vi "DataSummarizer.vi"() -> ()   [LabVIEW 2025]
uses:
  Controls/State.ctl
  ff876046-9b6a-4137-aed5-b25abd0cf997.vi
  <vilib>/Array/Sort 2D Array - Pop Stack.vi
  <vilib>/Array/Sort 2D Array - Push Stack.vi
  <vilib>/Utility/file.llb/Write Delimited Spreadsheet (string).vi
panel:
  out "output array":string[][](array[string])
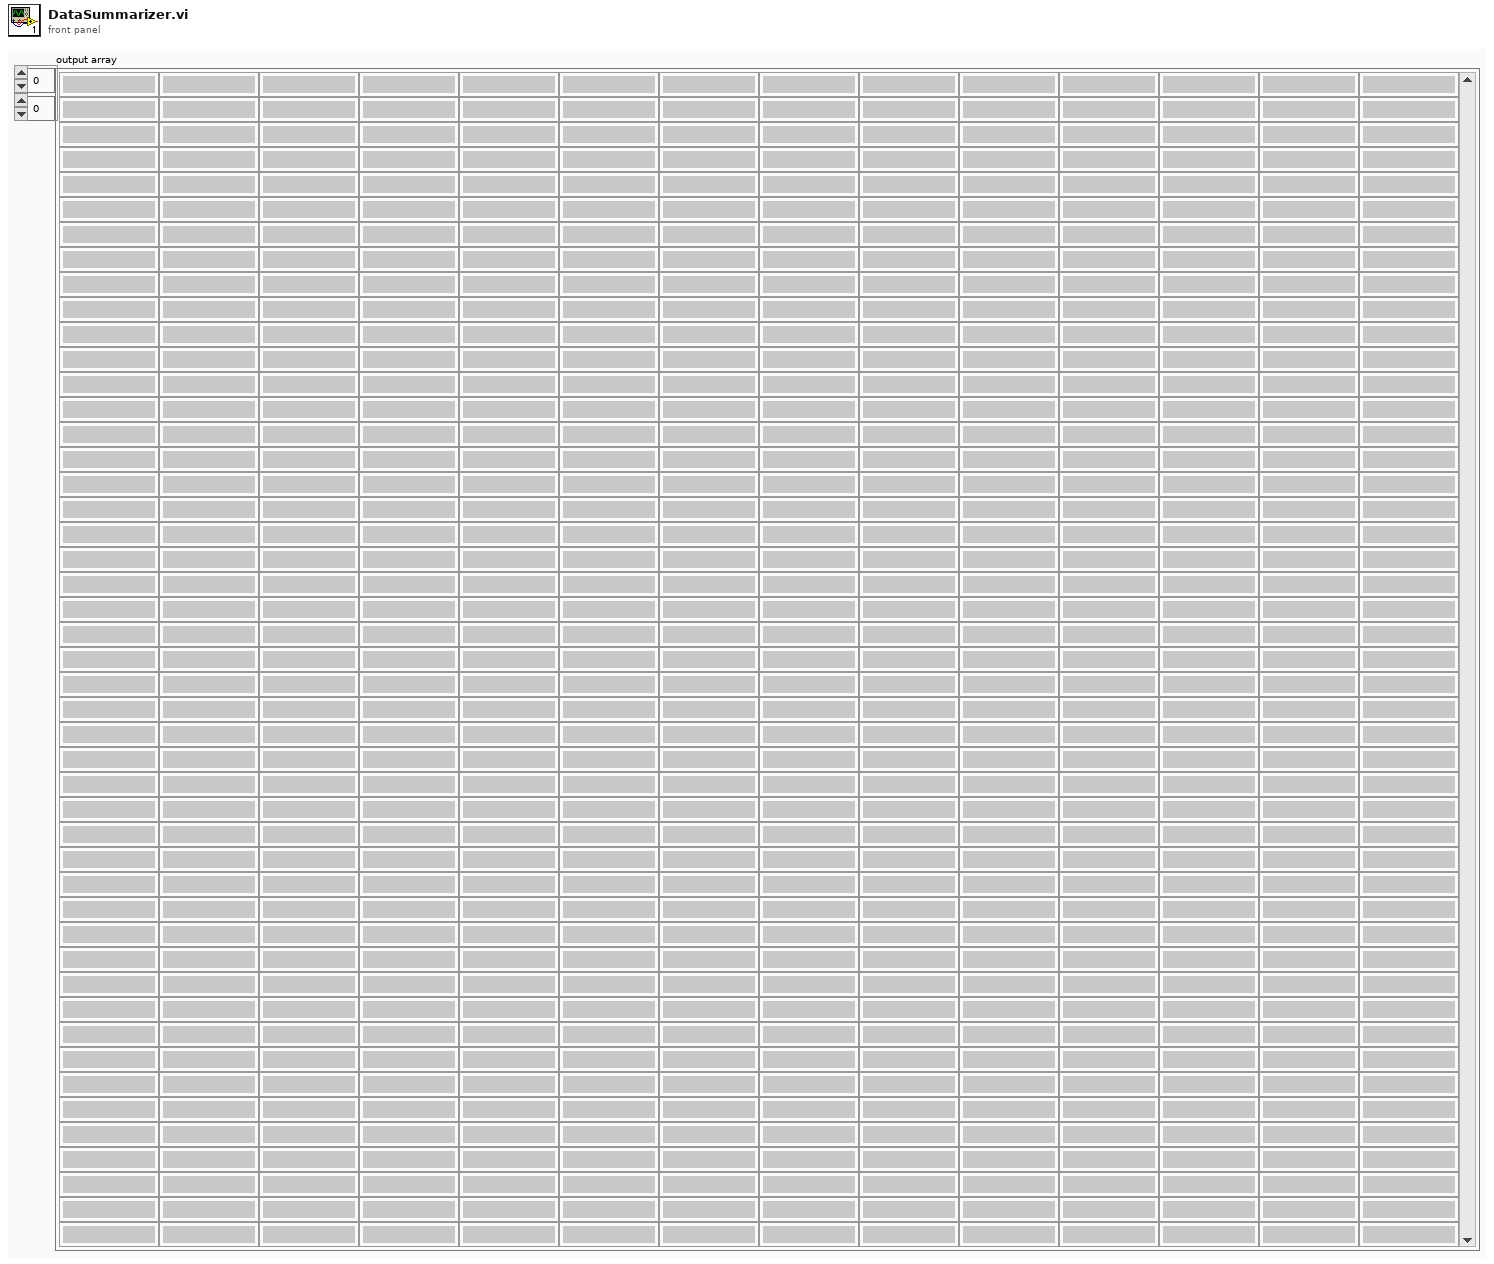
[diagram p1: front panel]
types:
  T1 = typedef "State.ctl" = enum16{"Init", "Idle", "Analyze", "End"}
  T2 = typedef "Dependand_Variables.ctl" = cluster{"Task Completion Times":dbl[], "TCT mean":dbl, "Error rate":i32, "Overshoots":i32[], "Overshoot  mean":dbl, "Overshoot times":dbl[], "Overshoot times mean":dbl, "targets out?":bool[], "No targets selected?":bool[], "No targets selected":i32}
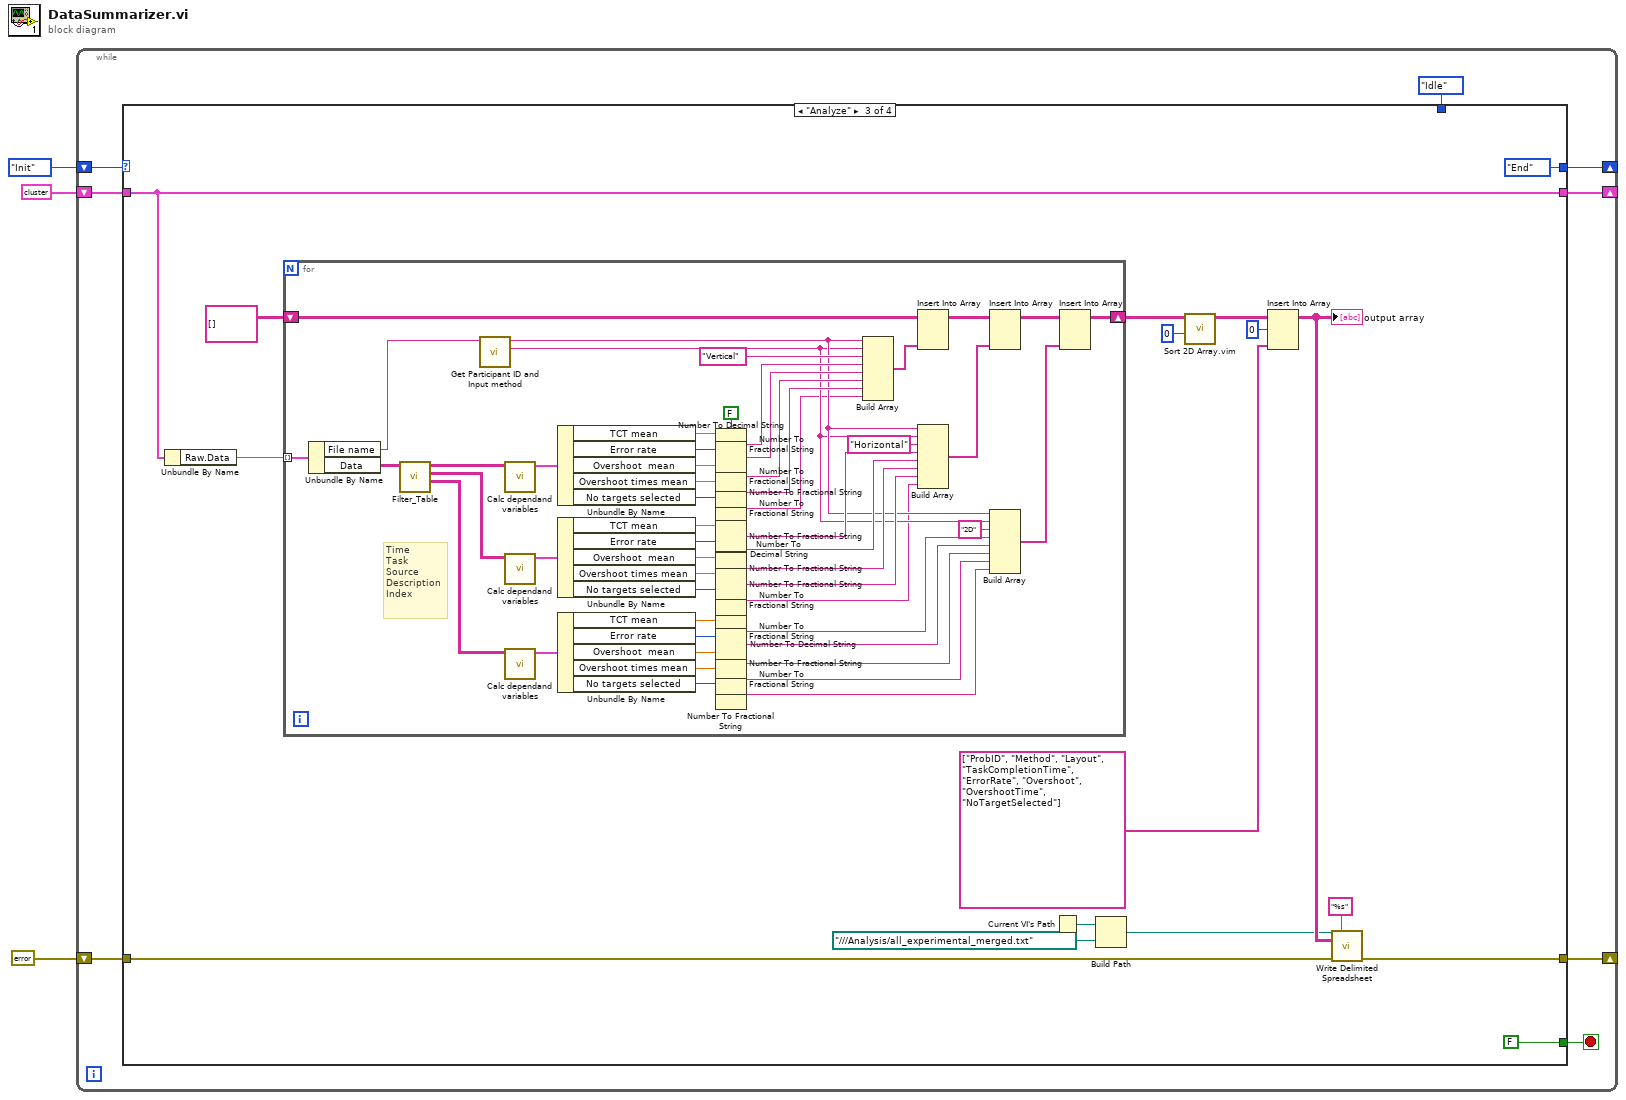
[diagram p0: block diagram]
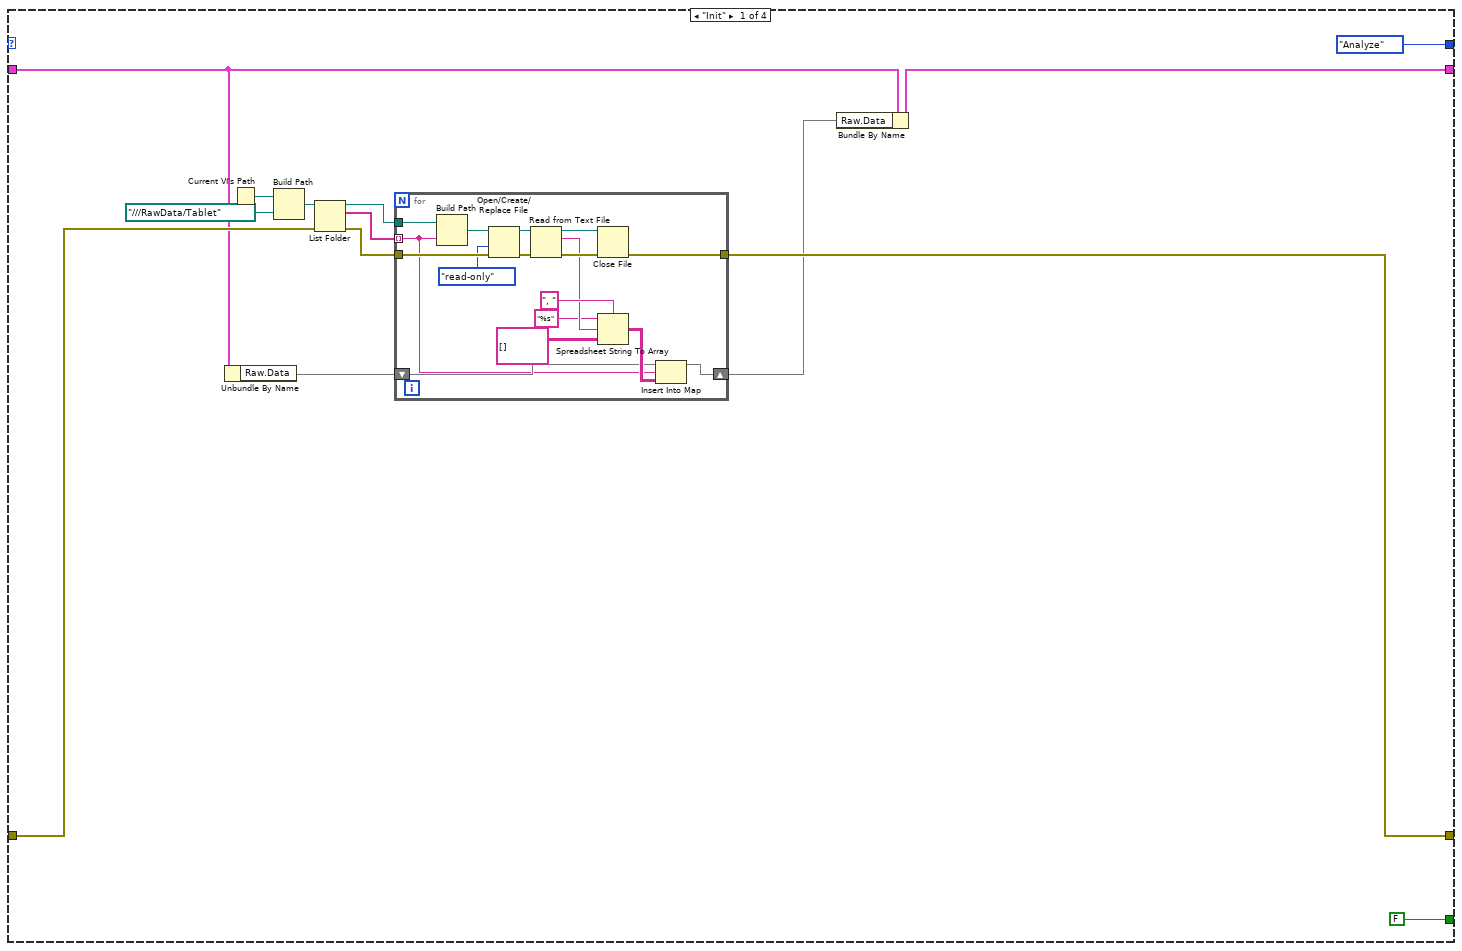
[diagram p2: hidden frame]
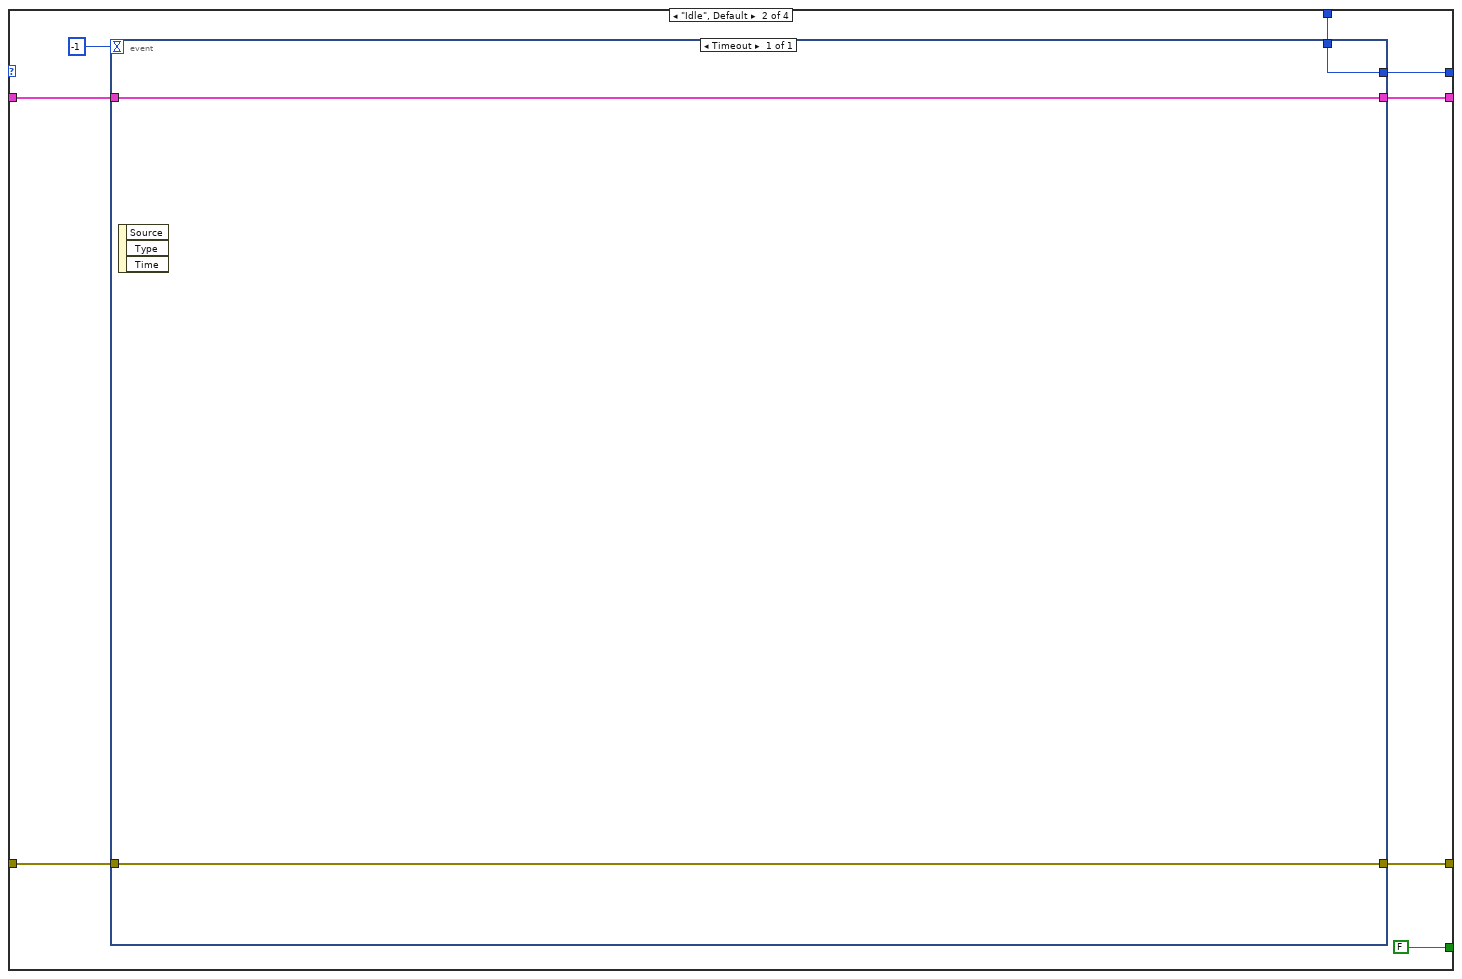
[diagram p3: hidden frame]
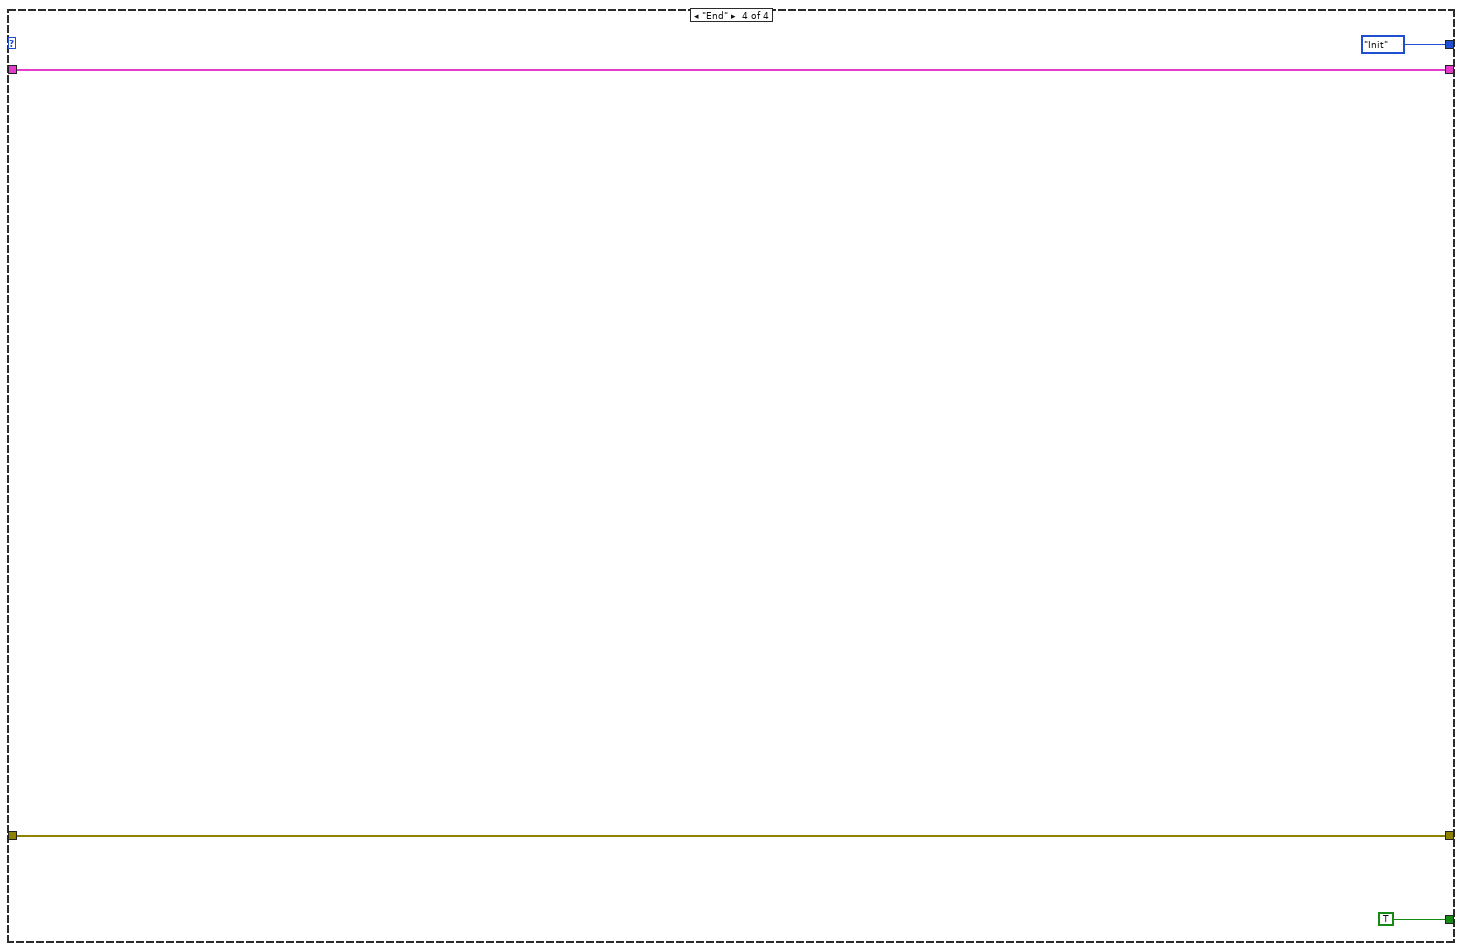
[diagram p4: hidden frame]
diagram:
  n1 = while {
    shift-right: [w9] -> _
    shift-left: errorcluster {"status"=FALSE, "code"=0, "source"=""} ("error constant") -> [w10]
    shift-right: [w8] -> _
    shift-left: State."Init" -> [w11]
    shift-right: [w5] -> _
    shift-left: cluster{"Raw.Data":map{string, string[][]}} {"Raw.Data"={}} -> [w6]
    stop <- w4 stop-if-true
    n2 = case shown="\"Analyze\"" w11 {
      tunnel: w10 -> [w22 w49 w58 w126]
      tunnel: [w21 w50 w57 w126] -> w9
      tunnel: [State."Analyze" w47 State."End" State."Init"] -> w8
      tunnel: State."Idle" -> [_ w46 _ _]
      tunnel: w6 -> [w18 w44 w69 w123]
      tunnel: [w19 w45 w69 w123] -> w5
      tunnel: [FALSE FALSE FALSE TRUE] -> w4
      frame "Init" {
        n3 = Unbundle By Name(w18) -> ("Raw.Data"=w17:map{string, string[][]})
        n4 = Current VI's Path() -> (path=w14:path)
        n5 = Build Path(base path=w14, name or relative path=path "../../../RawData/Tablet") -> (appended path=w12:path)
        n6 = List Folder(path=w12, error in=w22) -> (path out=w24:path, filenames=w25:string[], error out=w23:errorcluster)  [unwired: 2 in, 1 out]
        n7 = for {
          tunnel: w23 -> [w42]
          tunnel: w24 -> [w37]
          tunnel: w25 -> [w26] mode=indexing
          tunnel: [w30] -> w21
          shift-right: [w27] -> w16
          shift-left: w17 -> [w28]
          n8 = Build Path(base path=w37, name or relative path=w26) -> (appended path=w36:path)
          n9 = Open/Create/Replace File(file path (use dialog)=w36, error in=w42, access (0:read/write)=enum16{"read/write", "read-only", "write-only"}."read-only") -> (refnum out=w41:refnum<file>, error out=w40:errorcluster)  [unwired: 3 in, 1 out]
          n10 = Read from Text File(file (use dialog)=w41, error in=w40) -> (refnum out=w39:refnum<file>, text=w33:string, error out=w38:errorcluster)  [unwired: 2 in, 1 out]
          n11 = Close File(refnum=w39, error in=w38) -> (error out=w30:errorcluster)  [unwired: 1 out]
          n12 = Spreadsheet String To Array(delimiter (Tab)=", ", format string="%s", spreadsheet string=w33, array type (2D Dbl)=string[][] []) -> (array=w29:string[][])
          n13 = Insert Into Map(map in=w28, key=w26, value=w29) -> (map out=w27:map{string, string[][]})  [unwired: 2 out]
        }
        n14 = Bundle By Name(cluster=w18, "Raw.Data"=w16) -> (w19:cluster{"Raw.Data":map{string, string[][]}})
      }
      frame "Idle", Default {
        n15 = event shown="[0] Timeout" {
          selector: _ -> [_]
          dyn-events: _ -> [_]
          timeout: -1 -> [_]
          tunnel: [w53] -> w50
          tunnel: w49 -> [w53]
          tunnel: [w52] -> w47
          tunnel: w46 -> [w52]
          tunnel: [w51] -> w45
          tunnel: w44 -> [w51]
          event Timeout {
            n16 = event-data() -> ()  [unwired: 1 in, 3 out]
          }
        }
      }
      frame "Analyze" {
        n17 = Unbundle By Name(w69) -> ("Raw.Data"=w68:map{string, string[][]})
        n18 = for {
          tunnel: w68 -> [w120] mode=indexing
          shift-right: [w81] -> w62
          shift-left: string[][] [] -> [w100]
          w72 = FALSE ("use system decimal point (T)")
          # "Time\nTask\nSource\nDescription\nIndex"
          n19 = Unbundle By Name(w120) -> ("File name"=w80:string, "Data"=w119:string[][])
          n20 = call "Filter_Table.vi"("Table in"=w119) -> ("2D"=w122:string[][], "Horizontal"=w79:string[][], "Vertical"=w121:string[][])  [unwired: 8 in]
          n21 = call "Get Participant ID and Input method.vi"("File name"=w80) -> ("Input method"=w87:string, "Participant ID"=w88:string)  [unwired: 9 in]
          n22 = call "Calc dependand variables.vi"("Item Names"=w121) -> ("Dependand Variables"=w118:T2)  [unwired: 10 in]
          n23 = call "Calc dependand variables.vi"("Item Names"=w79) -> ("Dependand Variables"=w117:T2)  [unwired: 10 in]
          n24 = call "Calc dependand variables.vi"("Item Names"=w122) -> ("Dependand Variables"=w116:T2)  [unwired: 10 in]
          n25 = Unbundle By Name(w118) -> ("TCT mean"=w102:dbl, "Error rate"=w115:i32, "Overshoot  mean"=w114:dbl, "Overshoot times mean"=w113:dbl, "No targets selected"=w78:i32)
          n26 = Unbundle By Name(w117) -> ("TCT mean"=w112:dbl, "Error rate"=w111:i32, "Overshoot  mean"=w110:dbl, "Overshoot times mean"=w76:dbl, "No targets selected"=w75:i32)
          n27 = Unbundle By Name(w116) -> ("TCT mean"=w109:dbl, "Error rate"=w108:i32, "Overshoot  mean"=w107:dbl, "Overshoot times mean"=w106:dbl, "No targets selected"=w73:i32)
          n28 = Number To Fractional String(use system decimal point (T)=w72, number=w102) -> (F-format string=w105:string)  [unwired: 2 in]
          n29 = Number To Decimal String(number=w115) -> (decimal integer string=w104:string)  [unwired: 1 in]
          n30 = Number To Fractional String(use system decimal point (T)=w72, number=w114) -> (F-format string=w103:string)  [unwired: 2 in]
          n31 = Number To Fractional String(use system decimal point (T)=w72, number=w113) -> (F-format string=w101:string)  [unwired: 2 in]
          n32 = Number To Fractional String(use system decimal point (T)=w72, number=w78) -> (F-format string=w77:string)  [unwired: 2 in]
          n33 = Number To Fractional String(use system decimal point (T)=w72, number=w112) -> (F-format string=w93:string)  [unwired: 2 in]
          n34 = Number To Decimal String(number=w111) -> (decimal integer string=w92:string)  [unwired: 1 in]
          n35 = Number To Fractional String(use system decimal point (T)=w72, number=w110) -> (F-format string=w91:string)  [unwired: 2 in]
          n36 = Number To Fractional String(use system decimal point (T)=w72, number=w76) -> (F-format string=w90:string)  [unwired: 2 in]
          n37 = Number To Fractional String(use system decimal point (T)=w72, number=w75) -> (F-format string=w74:string)  [unwired: 2 in]
          n38 = Number To Fractional String(use system decimal point (T)=w72, number=w109) -> (F-format string=w86:string)  [unwired: 2 in]
          n39 = Number To Decimal String(number=w108) -> (decimal integer string=w85:string)  [unwired: 1 in]
          n40 = Number To Fractional String(use system decimal point (T)=w72, number=w107) -> (F-format string=w84:string)  [unwired: 2 in]
          n41 = Number To Fractional String(use system decimal point (T)=w72, number=w106) -> (F-format string=w83:string)  [unwired: 2 in]
          n42 = Number To Fractional String(use system decimal point (T)=w72, number=w73) -> (F-format string=w71:string)  [unwired: 2 in]
          n43 = Build Array(w88, w87, "Vertical" ("element"), w105, w104, w103, w101, w77) -> (w99:string[])
          n44 = Insert Into Array(array=w100, new element=w99) -> (w98:string[][])  [unwired: 2 in]
          n45 = Build Array(w88, w87, "Horizontal" ("element"), w93, w92, w91, w90, w74) -> (w95:string[])
          n46 = Insert Into Array(array=w98, new element=w95) -> (w97:string[][])  [unwired: 2 in]
          n47 = Build Array(w88, w87, "2D" ("element"), w86, w85, w84, w83, w71) -> (w82:string[])
          n48 = Insert Into Array(array=w97, new element=w82) -> (w81:string[][])  [unwired: 2 in]
        }
        n49 = Current VI's Path() -> (path=w56:path)
        n50 = Build Path(base path=w56, name or relative path=path "../../../Analysis/all_experimental_merged.txt") -> (appended path=w54:path)
        n51 = call "Sort 2D Array.vim"("index"=0, "2D array"=w62) -> ("sorted 2D array"=w61:string[][])  [unwired: 8 in, 1 out]
        n52 = Insert Into Array(array=w61, index (row)=0, new element=string[] ["ProbID", "Method", "Layout", "TaskCompletionTime", "ErrorRate", "Overshoot", "OvershootTime", "NoTargetSelected"]) -> (w59:string[][])  [unwired: 1 in]
        "output array" <- w59
        n53 = call-poly <vilib>:"Write Delimited Spreadsheet.vi"("file path (dialog if empty)"=w54, "format (%s)"="%s" ("format (%.3f)"), "2D data"=w59, "error in (no error)"=w58) -> ("error out"=w57:errorcluster)  [unwired: 10 in, 1 out]
      }
      frame "End" {
      }
    }
  }
